vi "NewtonsPSM_Retrieve_Sweep_FRA.vi"(0 "VISA session":refnum<visa-resource-name>, 11 "error in (no error)":errorcluster) -> (1 "Magnitude CH1":cluster{dbl[], dbl[]}(graph), 2 "Magnitude CH2":cluster{dbl[], dbl[]}(graph), 3 "dB":cluster{dbl[], dbl[]}(graph), 4 "dup VISA session":refnum<visa-resource-name>, 6 "Read Strings":string, 12 "Phase":cluster{dbl[], dbl[]}(graph), 13 "Delay":cluster{dbl[], dbl[]}(graph), 15 "error out":errorcluster)   [LabVIEW 2025, in "NewtonsPSM1735.lvlib"]
doc: "This VI readback the Datastores into the PPA2530."
uses:
  NewtonsPSM1735.lvlib
panel:
  out "Retrieving Finished":bool
  out "Nb of points":dbl
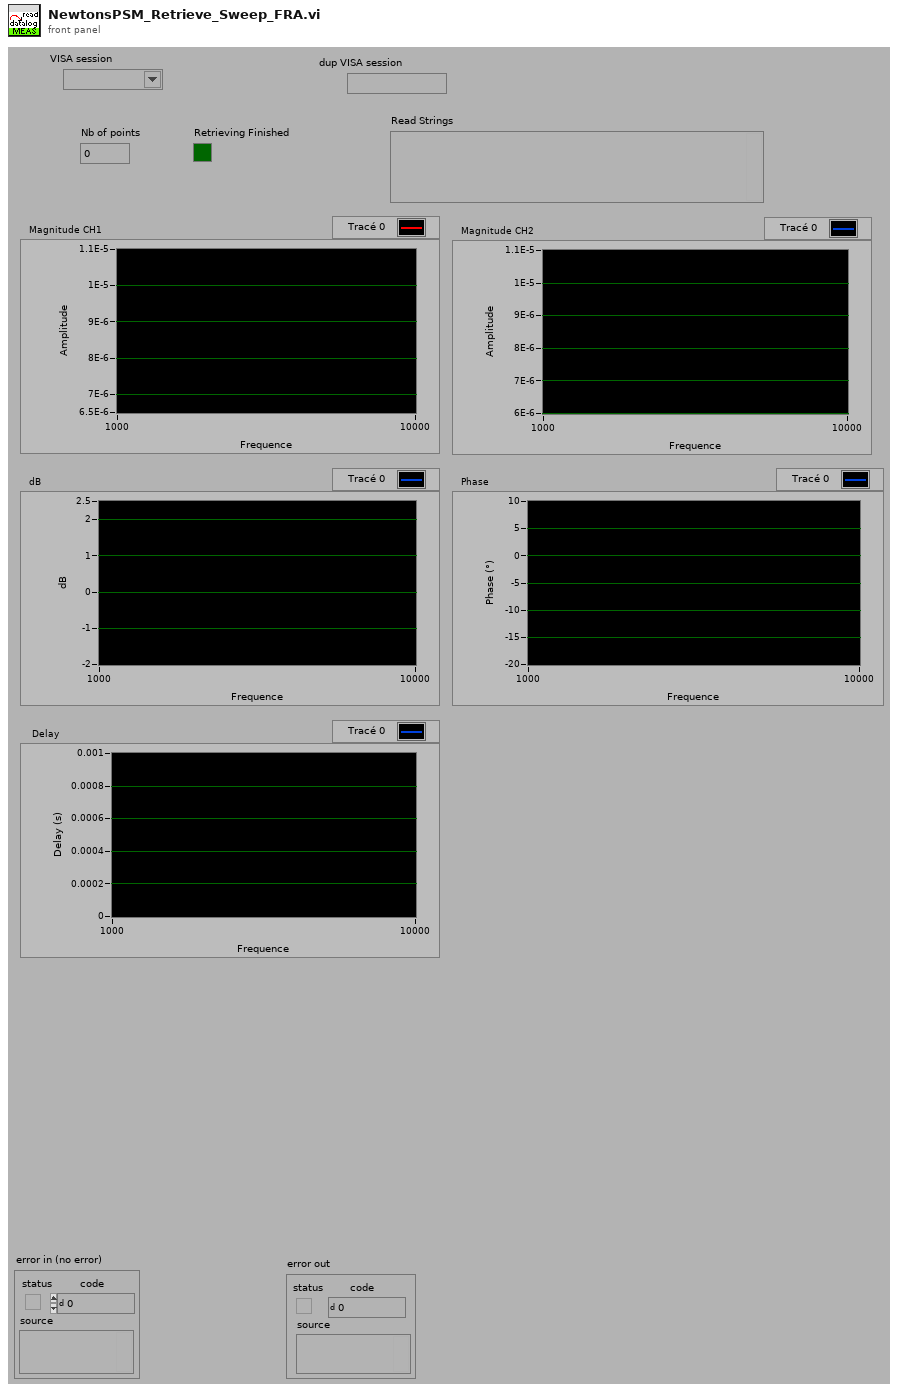
[diagram p1: front panel]
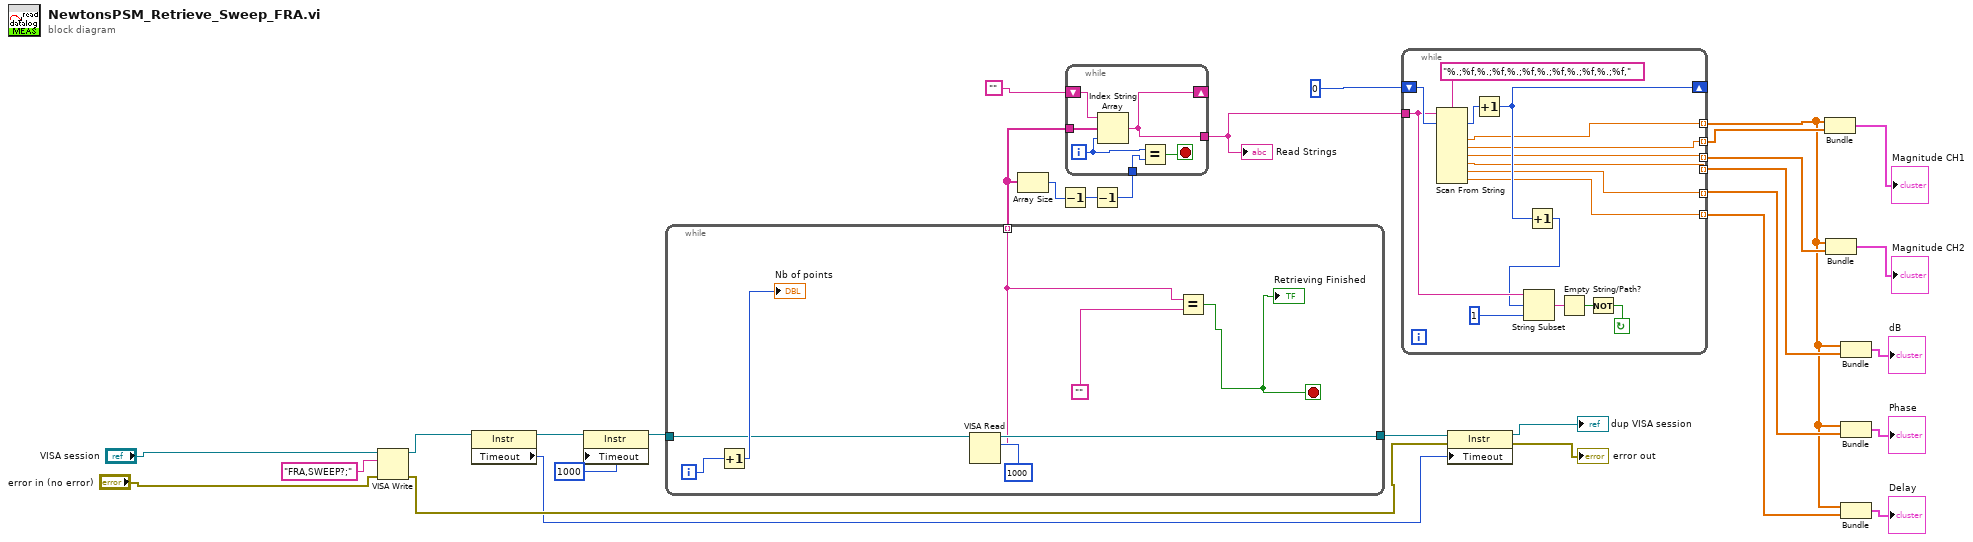
[diagram p0: block diagram]
diagram:
  n1 = VISA Write(VISA resource name="VISA session", write buffer="FRA,SWEEP?;" ("buffer à écrire"), error in (no error)="error in (no error)") -> (VISA resource name out=w3:refnum<visa-resource-name>, error out=w6:errorcluster)  [unwired: 1 out]
  n2 = property class="Instr"(reference=w3) -> (reference out=w4:refnum<visa-resource-name>, "Timeout"=w2:u32)  [unwired: 1 in, 1 out]
  n3 = property class="Instr"(reference=w4, "Timeout"=u32 1000 ("General Settings:Timeout Value")) -> (reference out=w10:refnum<visa-resource-name>)  [unwired: 1 in, 1 out]
  n4 = while {
    tunnel: [w36] -> w9
    tunnel: [w34] -> w29 mode=indexing
    tunnel: w10 -> [w32]
    i -> [w37]
    stop <- w31 stop-if-true
    n5 = Increment(x=w37) -> (x+1=→"Nb of points":i32)
    n6 = VISA Read(VISA resource name=w32, byte count=u32 1000 ("ÊÞ²Ä¶³ÝÄi0j")) -> (VISA resource name out=w36:refnum<visa-resource-name>, read buffer=w34:string)  [unwired: 1 in, 2 out]
    n7 = Equal?(x=w34, y="") -> (x = y?=w31:bool)
    "Retrieving Finished" <- w31
  }
  n8 = Array Size(array=w29) -> (size(s)=w27:i32)
  n9 = Decrement(x=w27) -> (x-1=w26:i32)
  n10 = Decrement(x=w26) -> (x-1=w25:i32)
  n11 = while {
    tunnel: w29 -> [w44]
    tunnel: [w40] -> w28
    tunnel: w25 -> [w41]
    shift-right: [w40] -> _
    shift-left: "" -> [w39]
    i -> [w42]
    stop <- w43 stop-if-true
    n12 = Index String Array(1:w42, 2:w44, 3:w39) -> (0:w40:string)
    n13 = Equal?(x=w42, y=w41) -> (x = y?=w43:bool)
  }
  "Read Strings" <- w28
  n14 = while {
    shift-left: 0 -> [w54]
    shift-right: [w52] -> _
    tunnel: [w48] -> w19 mode=indexing
    tunnel: w28 -> [w53]
    tunnel: [w49] -> w21 mode=indexing
    tunnel: [w50] -> w13 mode=indexing
    tunnel: [w47] -> w16 mode=indexing
    tunnel: [w46] -> w15 mode=indexing
    tunnel: [w45] -> w14 mode=indexing
    stop <- w57 continue-if-true
    n15 = Scan From String(format string="%.;%f,%.;%f,%.;%f,%.;%f,%.;%f,%.;%f,", input string=w53, initial scan location=w54) -> (offset past scan=w55:u32, output 1=w50:dbl, output 2=w49:dbl, output 3=w48:dbl, output 4=w47:dbl, output 5=w46:dbl, output 6=w45:dbl)  [unwired: 1 in, 8 out]
    n16 = Increment(x=w55) -> (x+1=w52:u32)
    n17 = Increment(x=w52) -> (x+1=w51:u32)
    n18 = String Subset(string=w53, offset (0)=w51, length (rest)=1) -> (substring=w59:string)
    n19 = Empty String/Path?(string/path=w59) -> (empty?=w58:bool)
    n20 = Not(x=w58) -> (.not. x?=w57:bool)
  }
  n21 = property class="Instr"(reference=w9, error in=w6, "Timeout"=w2) -> (reference out=→"dup VISA session":refnum<visa-resource-name>, error out=→"error out":errorcluster)
  n22 = Bundle(w13, w21) -> (→"Magnitude CH1":cluster{dbl[], dbl[]})  [unwired: 1 out]
  n23 = Bundle(w13, w19) -> (→"Magnitude CH2":cluster{dbl[], dbl[]})  [unwired: 1 out]
  n24 = Bundle(w13, w16) -> (→"dB":cluster{dbl[], dbl[]})  [unwired: 1 out]
  n25 = Bundle(w13, w15) -> (→"Phase":cluster{dbl[], dbl[]})  [unwired: 1 out]
  n26 = Bundle(w13, w14) -> (→"Delay":cluster{dbl[], dbl[]})  [unwired: 1 out]
